vi "Write Chassis Object.vi"(8 "error in":errorcluster, 10 "Chassis Information":T1 {"Modules"."Module Code" format="%.0x"; "Product ID" format="%.0x"}) -> (0 "error out":errorcluster, 3 "Chassis out":refnum<class "Chassis.lvclass">)   [LabVIEW 2015, in "SMI.lvlib" / "Chassis.lvclass"]
uses:
  Chassis.lvclass
  RT Management/Controls/ChassisInformation.ctl
  RT Management/RT Management.lvclass
  Module/Controls/ModuleInformation.ctl
  Module/Module.lvclass
panel:
  in  "Chassis in":refnum<class "Chassis.lvclass">
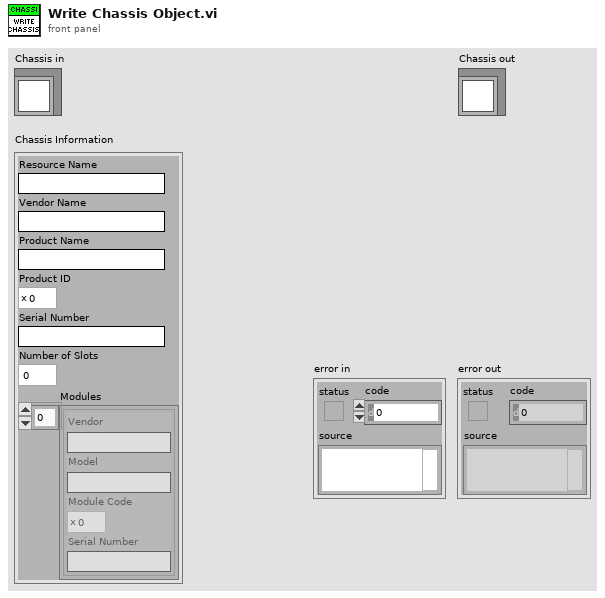
[diagram p1: front panel]
types:
  T1 = typedef "RT Management.lvlib/RT Management.lvclass/ChassisInformation.ctl" = cluster{"Resource Name":string, "Vendor Name":string, "Product Name":string, "Product ID":u32, "Serial Number":string, "Number of Slots":i32, "Modules":T2[]}
  T2 = typedef "SMI.lvlib/Module.lvclass/ModuleInformation.ctl" = cluster{"Vendor":string, "Model":string, "Module Code":u32, "Serial Number":string}
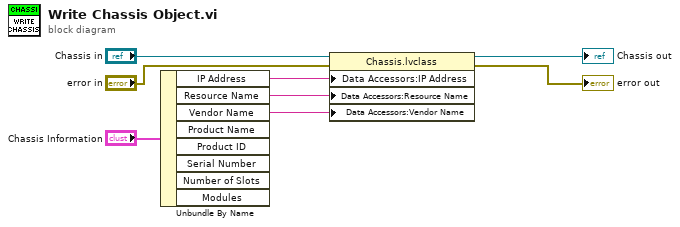
[diagram p0: block diagram]
diagram:
  n1 = Unbundle By Name("Chassis Information") -> ("IP Address"=w3:string, "Resource Name"=w2:string, "Vendor Name"=w1:string)  [unwired: 5 out]
  n2 = property class="Chassis.lvclass"(reference="Chassis in", error in="error in", "Data Accessors:IP Address"=w3, "Data Accessors:Resource Name"=w2, "Data Accessors:Vendor Name"=w1) -> (reference out=→"Chassis out":refnum<class "Chassis.lvclass">, error out=→"error out":errorcluster)
